vi "MAIN_merFISH_hybridization.vi"(0 "Data cluster":T1, 1 "queue valve":refnum<queue>, 2 "queue pump":refnum<queue>, 5 "Probe list":refnum<vi>, 7 "Valve H":u8(knob)=1 min=1 max=22 scale=1.0..22.0, 9 "variant":variant, 11 "error in":errorcluster, 12 "Hybridization manager Refnum":refnum<vi>, 13 "Valve Refnum":refnum<vi>, 14 "Valve position OUT Refnum":refnum<vi>) -> (4 "Next task":T2, 15 "error out":errorcluster)   [LabVIEW 2015]
uses:
  CONTROLS/Q_main_element.ctl
  CONTROLS/Q_VALVE_element.ctl
  CONTROLS/Q_PUMP_element.ctl
  GLOBAL/Global_ABORT.vi
  GLOBAL/Global_VALVE.vi
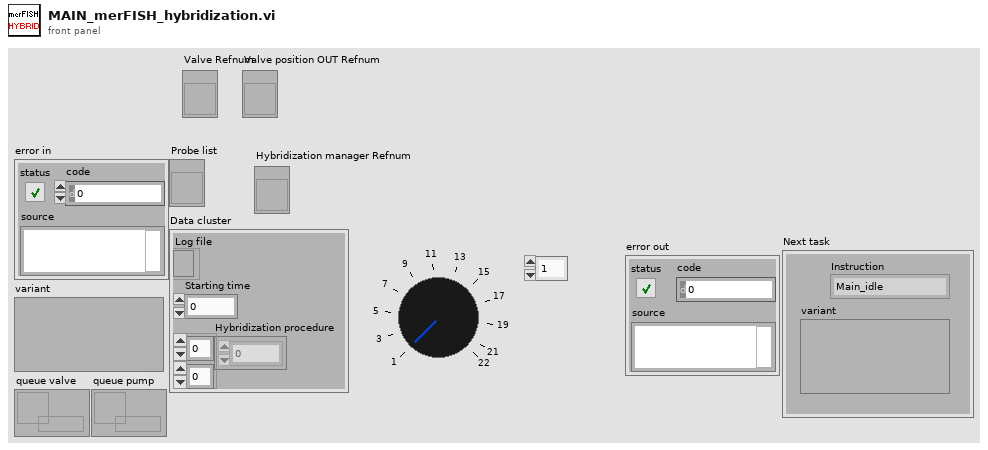
[diagram p1: front panel]
types:
  T1 = cluster{"Log file":refnum<file>, "Starting time":dbl, "Hybridization procedure":i32[][]}
  T2 = typedef "Q_main_element.ctl" = cluster{"variant":variant, "Instruction":enum16{"Main_idle", "Main_initialize", "Main_initialize_TDMS", "Main_initialize_Queue", "Main_error", "Main_DAQ_initialization_results", "Main_ASI_initialization_results", "Main_Piezo_initialization_results", "Main_Valve_initialization_results", "Main_Pump_initialization_results", "Main_CAMERA_initialization_results", "Main_FPGA_initialization_results", "Main_DAQ_error", "Main_ASI_error", "Main_Piezo_error", "Main_CAMERA_error", "Main_Valve_error", "Main_Pump_error", "Main_FPGA_error", "Main_start_acquiring", "Main_not_acquiring", "Main_acquiring", "Main_stop_acquiring", "Main_change_exposure", "Main_change_z_scan_parameters", "Main_define_ROI", "Main_define_mosaic", "Main_read_kinetic_time", "Main_cooler", "Main_read_temperature", "Main_save_XY", "Main_load_XY", "Main_discard_XY", "Main_move_to_XY", "Main_measure_QPD", "Main_autofocus_calibration", "Main_autofocus_initialization", "Main_autofocus_stop", "Main_save_PID", "Main_change_H_valve_position", "Main_two_way_valve", "Main_save_movie", "Main_init_single_scan", "Main_single_scan", "Main_stop_single_scan", "Main_merFISH_illumination_parameters", "Main_merFISH_buffer_probe_list", "Main_merFISH_injections_procedure", "Main_merFISH_save_setpoint", "Main_merFISH_DAPI_parameters", "Main_merFISH_Brightfield_parameters", "Main_merFISH_save_embryo_ROI", "Main_merFISH_init", "Main_merFISH_resume", "Main_merFISH_start_autofocus", "Main_merFISH_open_close_valve_merFISH", "Main_merFISH_open_close_valve_photobleaching", "Main_merFISH_hybridization", "Main_merFISH_move_to_ROI", "Main_merFISH_wait_stabilization", "Main_merFISH_move_to_REF", "Main_merFISH_scan", "Main_merFISH_photobleaching_injection", "Main_merFISH_photobleaching", "Main_merFISH_send_email", "Main_merFISH_close", "Main_STOP"}}
  T3 = cluster{"Pressure (mbar)":i32, "Volume (µl)":i32, "Flow rate (ul/s) ":i32}
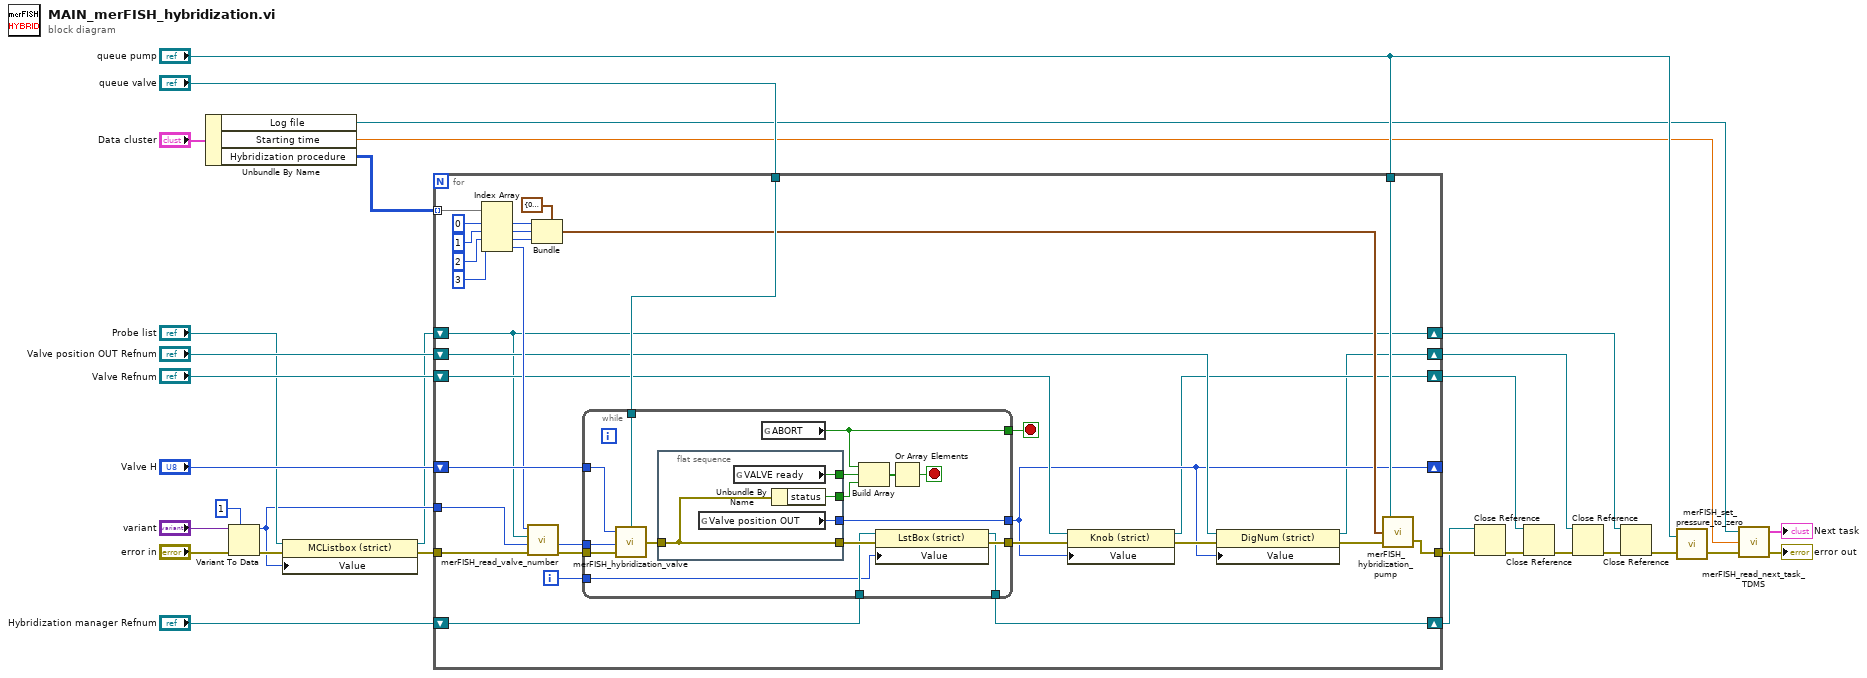
[diagram p0: block diagram]
diagram:
  n1 = Unbundle By Name("Data cluster") -> ("Log file"=w13:refnum<file>, "Starting time"=w12:dbl, "Hybridization procedure"=w11:i32[][])
  n2 = Variant To Data(error in="error in", type=1 ("Probe list"), Variant="variant") -> (data=w6:i32, error out=w8:errorcluster)
  n3 = property class="MCListbox (strict)"(reference="Probe list", error in=w8, "Value"=w6) -> (reference out=w4:refnum<vi>, error out=w5:errorcluster)
  n4 = for {
    tunnel: "queue valve" -> [w62]
    tunnel: "queue pump" -> [w55]
    tunnel: [w56] -> w19
    tunnel: w11 -> [w53] mode=indexing
    tunnel: w6 -> [w49]
    shift-right: [w35] -> _
    shift-left: "Valve H" -> [w48]
    tunnel: w5 -> [w42]
    shift-right: [w40] -> w18
    shift-left: "Hybridization manager Refnum" -> [w41]
    shift-right: [w33] -> w16
    shift-left: "Valve Refnum" -> [w38]
    shift-right: [w32] -> w14
    shift-left: "Valve position OUT Refnum" -> [w36]
    shift-right: [w31] -> w1
    shift-left: w4 -> [w31]
    i -> [w47]
    stop <- w50 stop-if-true
    n5 = Index Array(array=w53, index #1=0 ("index"), index #2=1 ("index"), index #3=2 ("index"), index #4=3 ("index")) -> (element #1=w58:i32, element #2=w57:i32, element #3=w44:i32, element #4=w45:i32)
    n6 = call "merFISH_read_valve_number.vi"("error in"=w42, "Probe #"=w49, "ProbeList Refnum"=w31, "Valve # IN"=w45) -> ("error out"=w52:errorcluster, "Valve # OUT"=w51:i32)  [unwired: 2 in]
    n7 = Bundle(cluster=T3 {"Pressure (mbar)"=0, "Volume (µl)"=0, "Flow rate (ul/s) "=0} ("input data cluster"), "Pressure (mbar)"=w58, "Volume (µl)"=w57, "Flow rate (ul/s)"=w44) -> (w54:T3)
    n8 = while {
      tunnel: w62 -> [w78]
      tunnel: w52 -> [w77]
      tunnel: [w64] -> w39
      tunnel: w51 -> [w75]
      tunnel: [w70] -> w50
      tunnel: w48 -> [w74]
      tunnel: [w73] -> w35
      tunnel: w47 -> [w65]
      tunnel: w41 -> [w66]
      tunnel: [w63] -> w40
      stop <- w72 stop-if-true
      n9 = call "merFISH_hybridization_valve.vi"("queue valve"=w78, "error in"=w77, "New position"=w75, "Valve H"=w74) -> ("error out"=w76:errorcluster)
      n10 = flat-sequence {
        tunnel: w76 -> [w80]
        tunnel: [w80] -> w67
        tunnel: [w82] -> w73
        tunnel: [w81] -> w71
        tunnel: [w79] -> w68
        frame #0 {
          n11 = global read "Global_VALVE.vi" "Valve position OUT"() -> (w82:u8)
          n12 = global read "Global_VALVE.vi" "VALVE ready"() -> (w81:bool)
          n13 = Unbundle By Name(w80) -> ("status"=w79:bool)
        }
      }
      n14 = global read "Global_ABORT.vi" "ABORT"() -> (w70:bool)
      n15 = Build Array(w70, w71, w68) -> (w69:bool[])
      n16 = property class="LstBox (strict)"(reference=w66, error in=w67, "Value"=w65) -> (reference out=w63:refnum<vi>, error out=w64:errorcluster)
      n17 = Or Array Elements(Boolean array=w69) -> (logical OR=w72:bool)
    }
    n18 = property class="Knob (strict)"(reference=w38, error in=w39, "Value"=w35) -> (reference out=w33:refnum<vi>, error out=w37:errorcluster)
    n19 = property class="DigNum (strict)"(reference=w36, error in=w37, "Value"=w35) -> (reference out=w32:refnum<vi>, error out=w34:errorcluster)
    n20 = call "merFISH_hybridization_pump.vi"("error in"=w34, "input data cluster"=w54, "queue pump"=w55) -> ("error out"=w56:errorcluster)  [unwired: 1 in]
  }
  n21 = Close Reference(reference=w18, error in (no error)=w19) -> (error out=w17:errorcluster)
  n22 = Close Reference(reference=w16, error in (no error)=w17) -> (error out=w15:errorcluster)
  n23 = Close Reference(reference=w14, error in (no error)=w15) -> (error out=w3:errorcluster)
  n24 = Close Reference(reference=w1, error in (no error)=w3) -> (error out=w2:errorcluster)
  n25 = call "merFISH_set_pressure_to_zero.vi"("error in"=w2, "queue pump"="queue pump") -> ("error out"=w30:errorcluster)  [unwired: 1 in]
  n26 = call "merFISH_read_next_task_TDMS.vi"("error in"=w30, "Starting time"=w12, "Log file"=w13) -> ("error out"=→"error out":errorcluster, "task"=→"Next task":T2)  [unwired: 1 in]
